vi "graph-density.vi"() -> ()   [LabVIEW 2014]
uses:
  <vilib>/Utility/file.llb/Read From Spreadsheet File (DBL).vi
panel:
  in  "Reduce Array Size":i32
  out "size(s) 2":i32
  out "XY Graph 2":cluster{dbl[], dbl[]}(graph)
  out "size(s)":i32
  out "XY Graph":cluster{dbl[], dbl[]}(graph)
  out "File":string
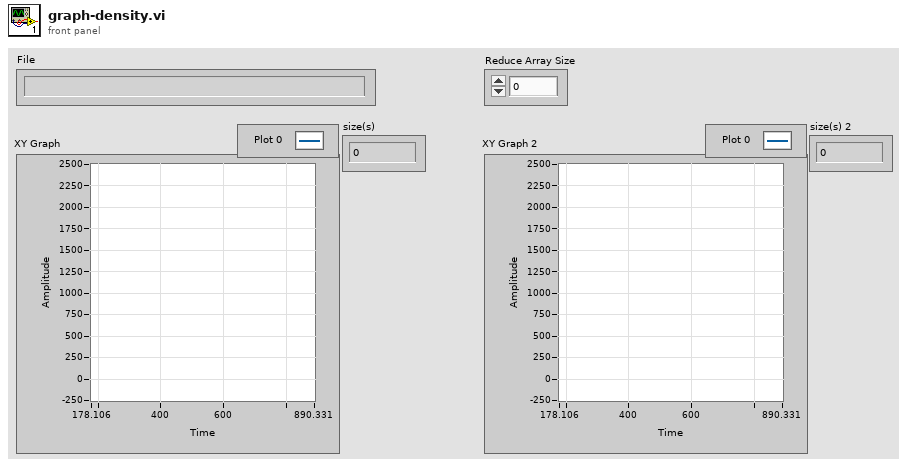
[diagram p1: front panel]
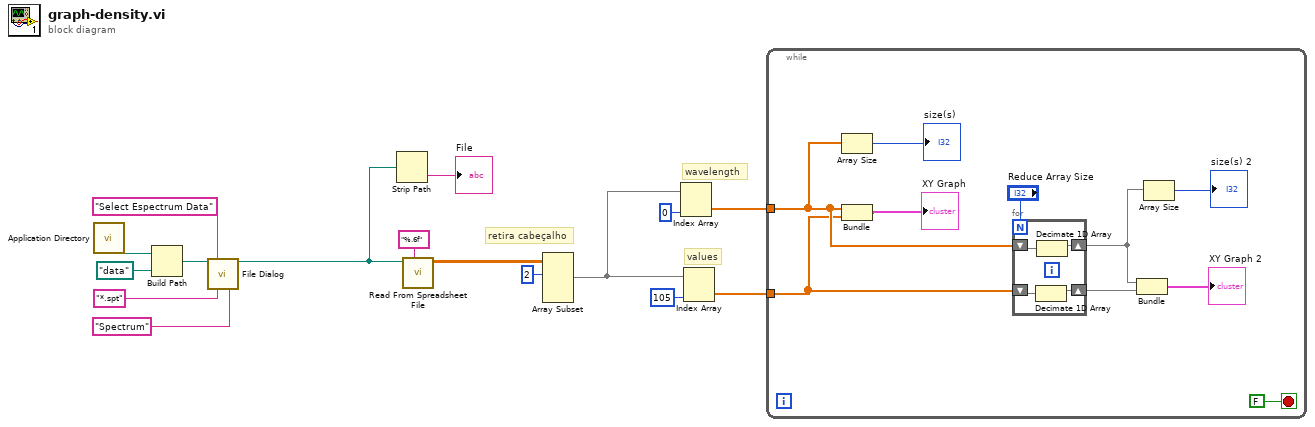
[diagram p0: block diagram]
diagram:
  # "values"
  # "wavelength"
  # "retira cabeçalho"
  n1 = call <vilib>:"Application Directory.vi"() -> ("Application Directory"=w7:path)
  n2 = Build Path(base path=w7, name or relative path=path "data") -> (appended path=w6:path)
  n3 = call "File Dialog"("start path"=w6, "prompt"="Select Espectrum Data", "pattern (all files)"="*.spt", "pattern label"="Spectrum") -> ("selected path"=w5:path)  [unwired: 8 in, 3 out]
  n4 = Strip Path(path=w5) -> (name=→"File":string)  [unwired: 1 out]
  n5 = call-poly <vilib>:"Read From Spreadsheet File.vi"("format (%.3f)"="%.6f", "file path (dialog if empty)"=w5) -> ("all rows"=w15:dbl[][])  [unwired: 5 in, 4 out]
  n6 = Array Subset(array=w15, index (row)=2 ("index")) -> (w3:dbl[][])  [unwired: 3 in]
  n7 = Index Array(array=w3, index (col)=0 ("disabled index (col)")) -> (element=w2:dbl[])  [unwired: 1 in]
  n8 = Index Array(array=w3, index (col)=105 ("disabled index (col)")) -> (element=w1:dbl[])  [unwired: 1 in]
  n9 = while {
    tunnel: w2 -> [w21]
    tunnel: w1 -> [w20]
    stop <- FALSE stop-if-true
    n10 = Array Size(array=w21) -> (size(s)=→"size(s)":i32)
    n11 = Bundle(w21, w20) -> (→"XY Graph":cluster{dbl[], dbl[]})  [unwired: 1 in]
    n12 = for {
      N: "Reduce Array Size" -> [_]
      shift-right: [w28] -> w19
      shift-left: w21 -> [w30]
      shift-right: [w27] -> w18
      shift-left: w20 -> [w29]
      n13 = Decimate 1D Array(w29) -> (w27:dbl[])  [unwired: 1 out]
      n14 = Decimate 1D Array(w30) -> (w28:dbl[])  [unwired: 1 out]
    }
    n15 = Bundle(w19, w18) -> (→"XY Graph 2":cluster{dbl[], dbl[]})  [unwired: 1 in]
    n16 = Array Size(array=w19) -> (size(s)=→"size(s) 2":i32)
  }
